vi "경로 (2).vi"() -> ()   [LabVIEW 2014]
panel:
  out "연결된 문자열":string
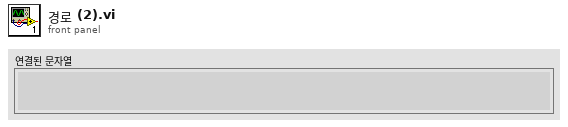
[diagram p1: front panel]
types:
  T1 = enum16{"open", "replace", "create", "open or create", "replace or create", "replace or create with confirmation"}
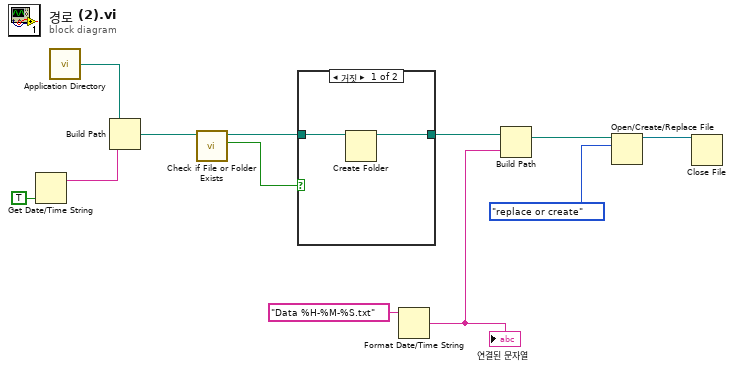
[diagram p0: block diagram]
diagram:
  n1 = Get Date/Time String(want seconds? (F)=TRUE ("초 보이기? (거짓)")) -> (date string=w1:string)  [unwired: 2 in, 1 out]
  n2 = call <vilib>:"Application Directory.vi"() -> ("Application Directory"=w2:path)
  n3 = Build Path(base path=w2, name or relative path=w1) -> (appended path=w10:path)
  n4 = call <vilib>:"Check if File or Folder Exists.vi"("path"=w10) -> ("file or folder exists?"=w9:bool, "dup path"=w8:path)  [unwired: 8 in, 1 out]
  n5 = case shown="거짓" w9 {
    tunnel: w8 -> [w14 w15]
    tunnel: [w13 w15] -> w7
    frame False {
      n6 = Create Folder(path (use dialog)=w14) -> (created path=w13:path)  [unwired: 2 in, 2 out]
    }
    frame True {
    }
  }
  n7 = Format Date/Time String(time format string (%c)="Data %H-%M-%S.txt" ("시간 포맷 문자열 (%c)")) -> (date/time string=w6:string)  [unwired: 2 in]
  "연결된 문자열" <- w6
  n8 = Build Path(base path=w7, name or relative path=w6) -> (appended path=w5:path)
  n9 = Open/Create/Replace File(file path (use dialog)=w5, operation (0:open)=T1."replace or create" ("동작(0:open)")) -> (refnum out=w3:refnum<file>)  [unwired: 4 in, 2 out]
  n10 = Close File(refnum=w3) -> ()  [unwired: 1 in, 2 out]
